vi "Fetch Single Record Single Channel(I16).vi"(5 "FIFO Type":enum16{"FPGA to Host FIFO (U64)", "Generic"}(ring), 7 "Timeout (s)":i32=5, 8 "error in":errorcluster, 11 "FPGA VI Reference In":refnum<k20>) -> (0 "error out":errorcluster, 2 "Acquired Data":i16[](array[numeric]), 3 "FPGA VI Reference Out":refnum<k20>)   [LabVIEW 2011]
uses:
  <userlib>/FlexRIO Host Library/FlexRIO Host API/Acquire/Fetch/Fetch Acquired Data (U64).vi
  <vilib>/Utility/error.llb/Error Cluster From Error Code.vi
  <vilib>/rvi/errors/niLvFpgaAdjustHostInterfaceError.vi
  <vilib>/rvi/interface/nirviReadWriteControl/nirviReadWriteControl.xnode
  NiFpgaLv.dll
  <vilib>/rvi/interface/Simulation/niFpgaSimulationCallBeginRW.vi
  <userlib>/FlexRIO Host Library/FlexRIO Host Library (User).lvlib
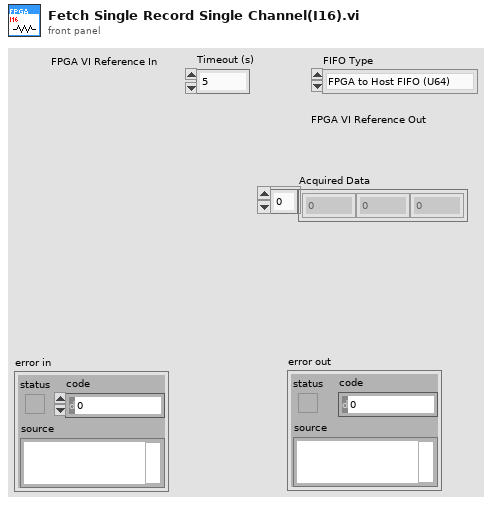
[diagram p1: front panel]
types:
  T1 = cluster{"Load Record Parameters?":bool, "Pre Trigger Samples":u16, "Samples per Record":u16, "Trigger Hold Off":u16, "Record Count":u16}
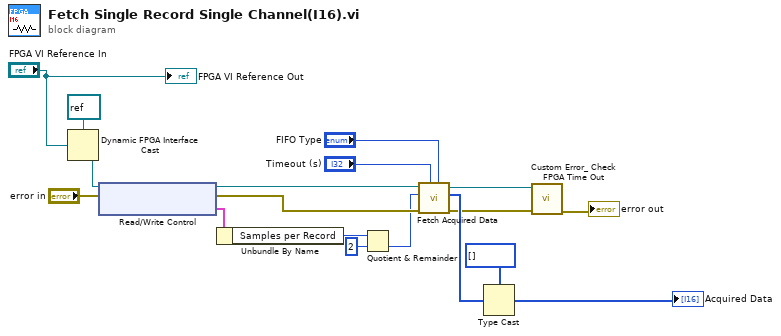
[diagram p0: block diagram]
diagram:
  n1 = Dynamic FPGA Interface Cast(Session In=refnum<k20> refnum ("Type"), Type="FPGA VI Reference In") -> (Session Out=w15:refnum<k20>)
  n2 = xnode "Read/Write Control"("FPGA VI Reference In"=w15, "error in"="error in") -> ("FPGA VI Reference Out"=w12:refnum<k20>, "error out"=w11:errorcluster, "Record Parameters"=w14:T1)
  n3 = Unbundle By Name(w14) -> ("Samples per Record"=w13:u16)
  n4 = Quotient & Remainder(x=w13, y=u16 2) -> (floor(x/y)=w2:u16)  [unwired: 1 out]
  n5 = call-poly <userlib>:"Fetch Acquired Data.vi"("FIFO Type"="FIFO Type", "Timeout (s)"="Timeout (s)", "error out"=w11, "Samples"=w2, "FPGA VI Reference In"=w12) -> ("error out"=w5:errorcluster, "Data"=w9:u64[], "FPGA VI Reference Out"=w6:refnum<k20>)  [unwired: 3 in, 1 out]
  n6 = Type Cast(type=i16[] [], x=w9) -> (*(type *) &x=→"Acquired Data":i16[])
  n7 = call <userlib>:"Custom Error_ Check FPGA Time Out.vi"("error in"=w5, "FPGA VI Reference In"=w6) -> ("error out"=→"error out":errorcluster)  [unwired: 8 in, 1 out]
  "FPGA VI Reference Out" <- "FPGA VI Reference In"
